vi "Get Raw Depth.vi"(8 "Error In":errorcluster, 11 "Index":i32) -> (0 "Error Out":errorcluster, 2 "Timestamp (ms)":u32, 3 "Raw Depth Data":u16[][](array[numeric]))   [LabVIEW 2011, in "LVH-Interface-for-Kinect.lvlib"]
uses:
  <vilib>/LabVIEW Hacker/LVH-Interface-for-Kinect/LVH-Interface-for-Kinect.lvlib
  <vilib>/LabVIEW Hacker/LVH-Interface-for-Kinect/Public/lib/freenect_sync.dll
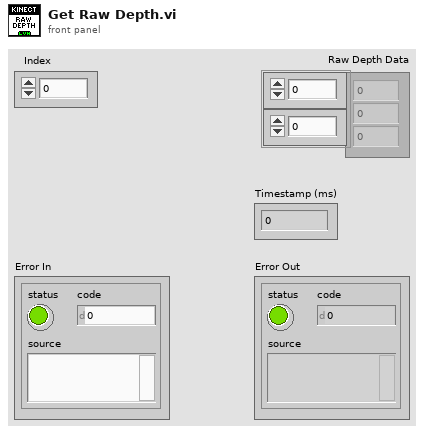
[diagram p1: front panel]
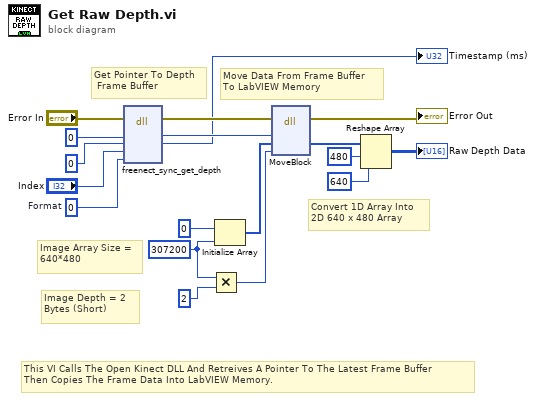
[diagram p0: block diagram]
diagram:
  w8 = u16 0  # Format
  w15 = 307200 ("dimension size")
  # "This VI Calls The Open Kinect DLL And Retreives A Pointer To The Latest Frame Buffer\nThen Copies The Frame Data Into LabVIEW Memory."
  # "Move Data From Frame Buffer\nTo LabVIEW Memory"
  # "Convert 1D Array Into \n2D 640 x 480 Array"
  # "Get Pointer To Depth\n Frame Buffer"
  # "Image Depth = 2 Bytes (Short)"
  # "Image Array Size = 640*480"
  n1 = dll-call lib="C:/Program Files (x86)/National Instruments/LabVIEW 2011/vi.lib/LabVIEW Hacker/LVH-Interface-for-Kinect/Public/lib/freenect_sync.dll" fn="freenect_sync_get_depth"(error in="Error In", "ptr"=i64 0, "timestamp"=u32 0, "index"="Index", "fmt"=w8) -> (error out=w17:errorcluster, "ptr"=w12:i64, "timestamp"=→"Timestamp (ms)":u32)  [unwired: 3 in, 3 out]
  n2 = Multiply(x=w15, y=2) -> (x*y=w13:i32)
  n3 = Initialize Array(u16 0 ("element"), w15) -> (w16:u16[])
  n4 = dll-call lib="LabVIEW" fn="MoveBlock"(error in=w17, "Address (Pointer)"=w12, "Destination"=w16, "Size"=w13) -> (error out=→"Error Out":errorcluster, "Destination"=w7:u16[])  [unwired: 4 in, 2 out]
  n5 = Reshape Array(w7, 480 ("dimension size"), 640 ("dimension size")) -> (→"Raw Depth Data":u16[][])
